vi "SubViTestCore.vi"   [LabVIEW 2014]
uses:
  <vilib>/rvi/Emulation/niFpgaGetClockAttributes.vi
  <vilib>/rvi/Emulation/niFpgaSctlEmulationGetInTimedLoop.vi
  <vilib>/rvi/Emulation/niFpgaEmulationReportErrorSimple.vi
  SubViTestGlobals.vi
  <vilib>/rvi/Emulation/niFpgaProcessEmulError.vi
  <vilib>/rvi/Emulation/niFpgaCriticalErrorInLSC.vi
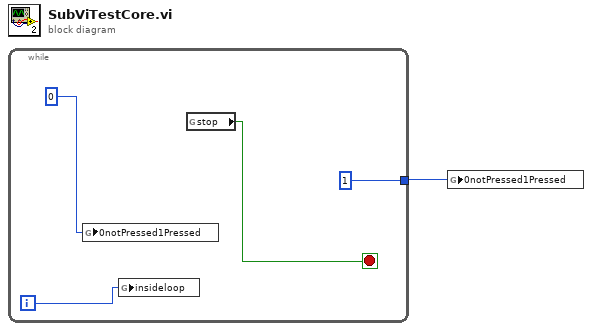
[diagram p0: block diagram]
diagram:
  n1 = while {
    tunnel: [i16 1] -> w1
    i -> [w3]
    stop <- w2 stop-if-true
    n2 = global write "SubViTestGlobals.vi" "0notPressed1Pressed"(i16 0) -> ()
    n3 = global write "SubViTestGlobals.vi" "insideloop"(w3) -> ()
    n4 = global read "SubViTestGlobals.vi" "stop"() -> (w2:bool)
  }
  n5 = global write "SubViTestGlobals.vi" "0notPressed1Pressed"(w1) -> ()
